vi "规范小时时间戳.vi"(11 "字符串":string) -> (3 "result string":string)   [LabVIEW 2016]
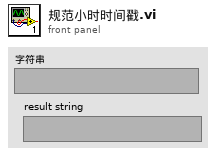
[diagram p1: front panel]
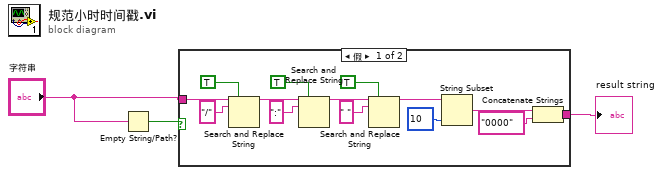
[diagram p0: block diagram]
diagram:
  n1 = Empty String/Path?(string/path="字符串") -> (empty?=w1:bool)
  n2 = case shown="假" w1 {
    tunnel: "字符串" -> [w8 w18]
    tunnel: [w7 w18] -> w3
    frame False {
      n3 = Search and Replace String(replace all?=TRUE ("替换全部？(F)"), input string=w8, search string="/" ("搜索字符串")) -> (result string=w11:string)  [unwired: 5 in, 3 out]
      n4 = Search and Replace String(replace all?=TRUE ("替换全部？(F)"), input string=w11, search string=":" ("搜索字符串")) -> (result string=w10:string)  [unwired: 5 in, 3 out]
      n5 = Search and Replace String(replace all?=TRUE ("替换全部？(F)"), input string=w10, search string=" " ("搜索字符串")) -> (result string=w14:string)  [unwired: 5 in, 3 out]
      n6 = String Subset(string=w14, length (rest)=10 ("长度（剩余）")) -> (substring=w16:string)  [unwired: 1 in]
      n7 = Concatenate Strings(w16, "0000" ("字符串")) -> (w7:string)
    }
    frame True {
    }
  }
  "result string" <- w3
